vi "MSScript_SubVI_RedMarkExpSection.vi"(6 "Enable":bool, 9 "Expression.Section":cluster{"STR":string, "Start":i32}, 10 "CMNT":cluster{"Start":u32, "End":u32}[](array[cluster]), 11 "String in":refnum<vi>) -> ()   [LabVIEW 2018, in "MSScript.lvclass"]
uses:
  MSScript.lvclass
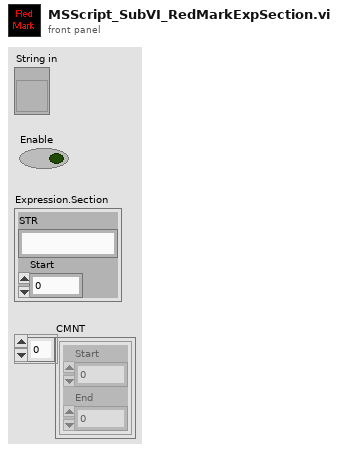
[diagram p1: front panel]
types:
  T1 = cluster{"Colour":u32, "Italic":bool, "Bold":bool}
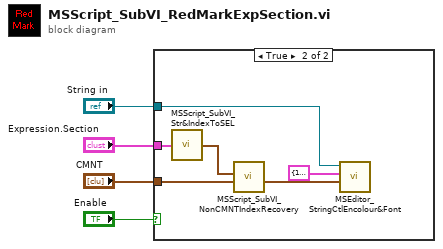
[diagram p0: block diagram]
diagram:
  n1 = case shown="True" "Enable" {
    tunnel: "CMNT" -> [_ w9]
    tunnel: "String in" -> [_ w8]
    tunnel: "Expression.Section" -> [_ w7]
    frame False {
    }
    frame True {
      n2 = call "MSScript_SubVI_Str&IndexToSEL.vi"("Name string"=w7) -> ("SEL"=w6:cluster{"Start":u32, "End":u32}[])
      n3 = call "MSScript_SubVI_NonCMNTIndexRecovery.vi"("SEL of CMNT"=w9, "NonCMNT.SEL"=w6) -> ("RecoverySEL"=w10:cluster{"Start":u32, "End":u32}[])  [unwired: 5 in]
      n4 = call "MSEditor_StringCtlEncolour&Font.vi"("SELs"=w10, "TextProperties"=T1 {"Colour"=16711680, "Italic"=FALSE, "Bold"=FALSE}, "String ctl ref"=w8) -> ()  [unwired: 7 in, 2 out]
    }
  }
